vi "Configure CIC Decimator.vi"(7 "index":i32, 8 "error in":errorcluster, 10 "decimation":i32, 11 "fpga session in":refnum<k20>) -> (0 "error out":errorcluster, 3 "fpga session out":refnum<k20>)   [LabVIEW 2017, in "Lock-In Amplifier Example Host.lvlib"]
uses:
  Lock-In Amplifier Example Host.lvlib
  fpga type.ctl
  <vilib>/Utility/error.llb/Error Cluster From Error Code.vi
  <vilib>/rvi/errors/niLvFpgaAdjustHostInterfaceError.vi
  <vilib>/rvi/interface/nirviReadWriteControl/nirviReadWriteControl.xnode
  <vilib>/ErrorRing/Error Ring.xnode
  NiFpgaLv.dll
  <vilib>/rvi/interface/Simulation/niFpgaSimulationCallBeginRW.vi
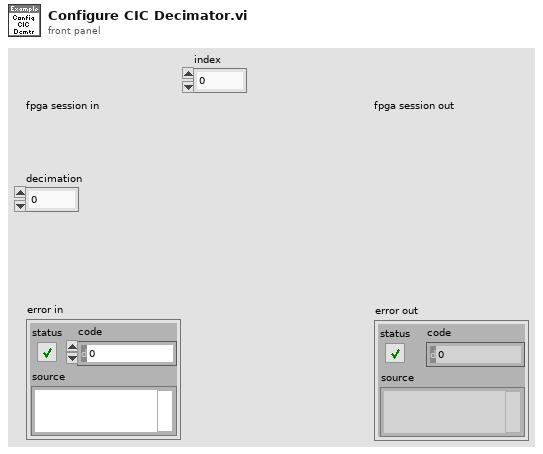
[diagram p1: front panel]
types:
  T1 = typedef "Lock-In Amplifier Example Host.lvlib/fpga type.ctl" = refnum<k20>
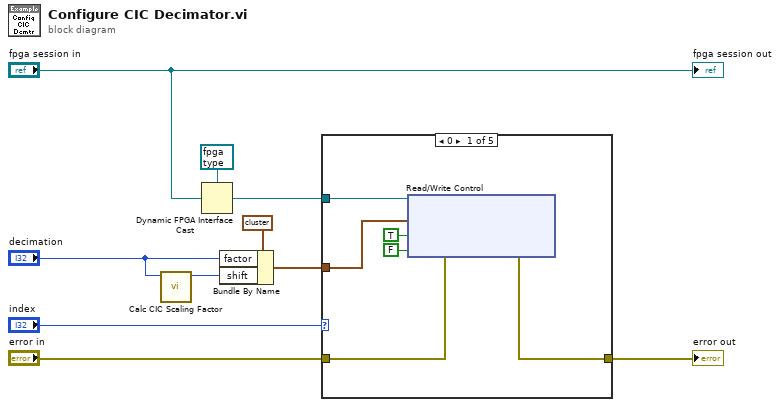
[diagram p0: block diagram]
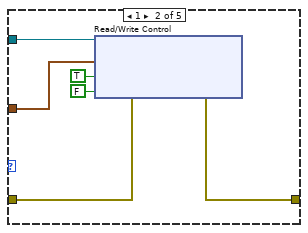
[diagram p2: hidden frame]
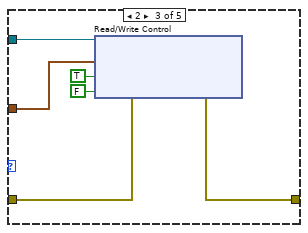
[diagram p3: hidden frame]
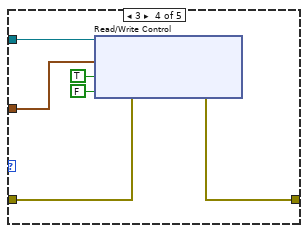
[diagram p4: hidden frame]
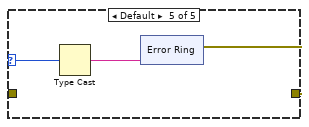
[diagram p5: hidden frame]
diagram:
  n1 = call "Calc CIC Scaling Factor.vi"("M"="decimation") -> ("shift"=w2:i32)  [unwired: 10 in]
  n2 = Dynamic FPGA Interface Cast(Session In=T1 refnum ("fpga type"), Type="fpga session in") -> (Session Out=w4:T1)
  n3 = Bundle By Name(cluster=cluster{"factor":fxp<+,16,16>, "shift":i16} {"factor"=0.0, "shift"=0} ("ai.cic config 0"), "factor"="decimation", "shift"=w2) -> (w1:cluster{"factor":fxp<+,16,16>, "shift":i16})
  n4 = case shown="0" "index" {
    selector: "index" -> [_ _ _ _ w37]
    tunnel: w4 -> [w16 w22 w28 w34 _]
    tunnel: w1 -> [w15 w21 w27 w33 _]
    tunnel: "error in" -> [w12 w18 w24 w30 _]
    tunnel: [w11 w17 w23 w29 w35] -> w7
    frame 0 {
      n5 = xnode "Read/Write Control"("FPGA VI Reference In"=w16, "error in"=w12, "lock-in.cic config 0"=w15, "lock-in.cic config valid 0"=TRUE ("ai.cic config valid 0"), "lock-in.cic config valid 0"=FALSE ("ai.cic config valid 0")) -> ("error out"=w11:errorcluster)  [unwired: 1 out]
    }
    frame 1 {
      n6 = xnode "Read/Write Control"("FPGA VI Reference In"=w22, "error in"=w18, "lock-in.cic config 1"=w21, "lock-in.cic config valid 1"=TRUE ("ai.cic config valid 0"), "lock-in.cic config valid 1"=FALSE ("ai.cic config valid 0")) -> ("error out"=w17:errorcluster)  [unwired: 1 out]
    }
    frame 2 {
      n7 = xnode "Read/Write Control"("FPGA VI Reference In"=w28, "error in"=w24, "lock-in.cic config 2"=w27, "lock-in.cic config valid 2"=TRUE ("ai.cic config valid 0"), "lock-in.cic config valid 2"=FALSE ("ai.cic config valid 0")) -> ("error out"=w23:errorcluster)  [unwired: 1 out]
    }
    frame 3 {
      n8 = xnode "Read/Write Control"("FPGA VI Reference In"=w34, "error in"=w30, "lock-in.cic config 3"=w33, "lock-in.cic config valid 3"=TRUE ("ai.cic config valid 0"), "lock-in.cic config valid 3"=FALSE ("ai.cic config valid 0")) -> ("error out"=w29:errorcluster)  [unwired: 1 out]
    }
    frame Default {
      n9 = Type Cast(x=w37) -> (*(type *) &x=w36:string)  [unwired: 1 in]
      n10 = xnode "Error Ring"("parameter 0"=w36) -> ("error out"=w35:errorcluster)
    }
  }
  "error out" <- w7
  "fpga session out" <- "fpga session in"
